vi "Control Power by Position.vi"(7 "Position":u32, 8 "error in (no error)":errorcluster, 10 "Power On?":bool, 11 "Driver Test in":refnum<class "Driver Test.lvclass">) -> (0 "error out":errorcluster)   [LabVIEW 2015, in "Driver Test.lvclass"]
doc: "Switch <b>Position</b> to <b>Power On?</b> state using fixture config defined switch routing."
uses:
  Driver Test.lvclass
  CBTF Applications/Driver Board Testing/Main/Application/Application/Class/typedefs/Instrument Selector -- Enum.ctl
  Classes/Instruments/Relay Control/Switch Executive/Switch Executive.lvclass
  CBTF Applications/Driver Board Testing/Main/Application/Application/Class/Driver Board Test.lvclass
  Test Class/Test Class.lvclass
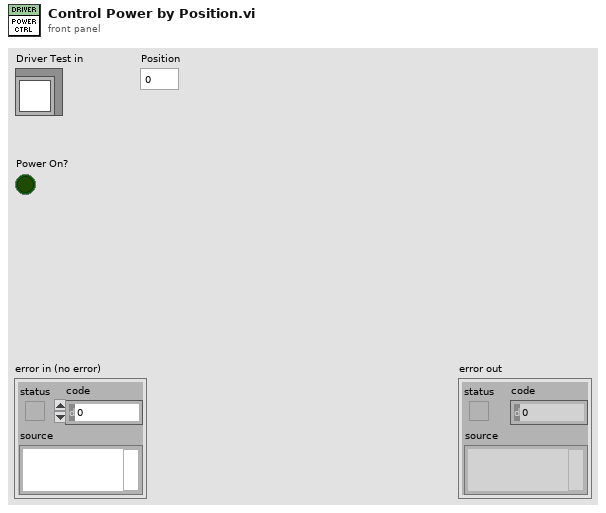
[diagram p1: front panel]
types:
  T1 = typedef "Driver Board Test.lvlib/Driver Board Test.lvclass/Instrument Selector -- Enum.ctl" = enum16{"ACPS1", "ACPS2", "DCPS1", "DCPS2", "DCPS3", "DCLoad1", "DCLoad2", "DPM1", "DPM2", "Switch1", "PXI1Slot2", "PXI1Slot3", "cDAQ1Mod5", "cDAQ1Mod6", "cDAQ1Mod7", "cDAQ1Mod8", "cDAQ1Mod1", "cDAQ1Mod2", "cDAQ1Mod3", "cDAQ1Mod4", "cDAQ2Mod1", "cDAQ2Mod2", "cDAQ2Mod3", "cDAQ2Mod4"}
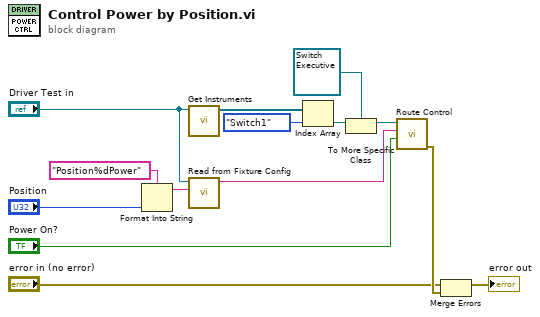
[diagram p0: block diagram]
diagram:
  n1 = Format Into String(format string="Position%dPower", "Position") -> (resulting string=w7:string)  [unwired: 2 in, 1 out]
  n2 = call "Get Instruments.vi"("Test Class in"="Driver Test in") -> ("Instruments"=w4:refnum<class "Instrument.lvclass">[])  [unwired: 9 in, 1 out]
  n3 = call-dynamic "Read from Fixture Config.vi"("Key"=w7, "Test Class in"="Driver Test in") -> ("Instrument Info"=w6:string)  [unwired: 8 in, 1 out]
  n4 = Index Array(array=w4, index=Instrument_Selector_--_Enum."Switch1" ("Instrument")) -> (element=w11:refnum<class "Instrument.lvclass">)
  n5 = To More Specific Class(target class=refnum<class "Switch Executive.lvclass"> refnum ("Switch Executive.lvlib:Switch Executive.lvclass"), reference=w11) -> (specific class reference=w13:refnum<class "Switch Executive.lvclass">)  [unwired: 1 in, 1 out]
  n6 = call-dynamic "Route Control.vi"("Connect (False)"="Power On?", "Route Name"=w6, "Switch Executive in"=w13) -> ("error out"=w14:errorcluster)  [unwired: 7 in, 1 out]
  n7 = Merge Errors("error in (no error)", w14) -> (→"error out":errorcluster)
